vi "Add Timestamp to DB.vi"(8 "error in (no error)":errorcluster, 10 "Timestamp":T1, 11 "TimeStamper in":refnum<class "TimeStamper.lvclass">) -> (0 "error out":errorcluster, 3 "TimeStamper out":refnum<class "TimeStamper.lvclass">)   [LabVIEW 2011, in "TimeStamper.lvclass"]
uses:
  TimeStamper.lvclass
  <vilib>/addons/database/NI_Database_API.lvlib
  AcquistionObject/AcquistionObject.lvclass
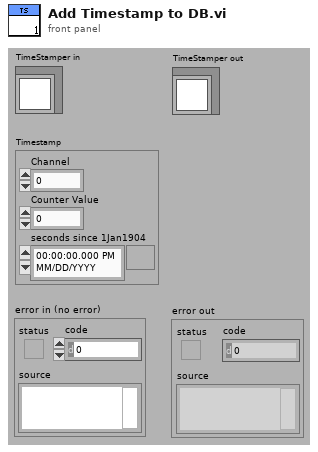
[diagram p1: front panel]
types:
  T1 = cluster{"Channel":i32, "Counter Value":u32, "seconds since 1Jan1904":timestamp}
  T2 = cluster{"setup":u8, "subject_id":u64, "session_start_time":dbl, "channel":u64, "counter":u64, "time":u64}
  T3 = typedef "NI_Database_API.lvlib/Conn ObjectReference.ctl" = refnum<k1>
  T4 = typedef "SessionPrimary.ctl" = cluster{"setup":u8, "subject_id":i32, "session_start_time":dbl}
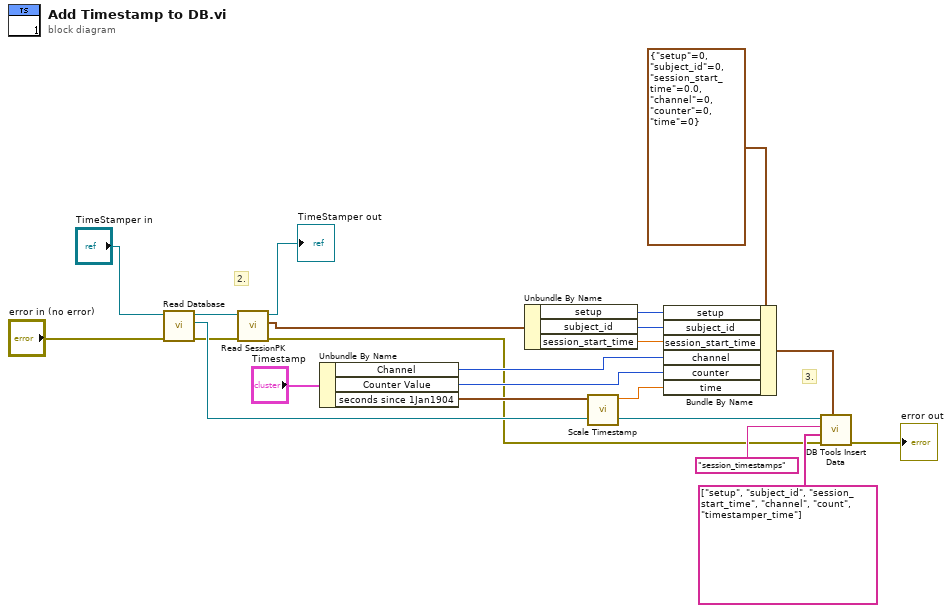
[diagram p0: block diagram]
diagram:
  # "2."
  # "3."
  n1 = call-dynamic "Read Database.vi"("error in (no error)"="error in (no error)", "AcquistionObject in"="TimeStamper in") -> ("error out"=w5:errorcluster, "reference"=w16:T3, "AcquistionObject out"=w2:refnum<class "TimeStamper.lvclass">)  [unwired: 7 in]
  n2 = call-dynamic "Read SessionPK.vi"("error in (no error)"=w5, "TimeStamper in"=w2) -> ("error out"=w4:errorcluster, "SessionPK"=w3:T4, "TimeStamper out"=→"TimeStamper out":refnum<class "TimeStamper.lvclass">)  [unwired: 7 in]
  n3 = Unbundle By Name("Timestamp") -> ("Channel"=w10:i32, "Counter Value"=w9:u32, "seconds since 1Jan1904"=w8:timestamp)
  n4 = Unbundle By Name(w3) -> ("setup"=w19:u8, "subject_id"=w18:i32, "session_start_time"=w6:dbl)
  n5 = call "Scale Timestamp.vi"("Time Stamp"=w8) -> ("Scaled timestamp"=w7:dbl)  [unwired: 10 in]
  n6 = Bundle By Name(cluster=T2 {"setup"=0, "subject_id"=0, "session_start_time"=0.0, "channel"=0, "counter"=0, "time"=0} ("Cluster"), "setup"=w19, "subject_id"=w18, "session_start_time"=w6, "channel"=w10, "counter"=w9, "time"=w7) -> (w17:T2)
  n7 = call <vilib>:"DB Tools Insert Data.vi"("data"=w17, "error in (no error)"=w4, "columns"=string[] ["setup", "subject_id", "session_start_time", "channel", "count", "timestamper_time"], "table"="session_timestamps", "connection reference"=w16) -> ("error out"=→"error out":errorcluster)  [unwired: 5 in, 1 out]
